vi "angle2DutyCycle.vi"(1 "Steering Angle":dbl min=-21.0 max=21.0 step=1.0) -> (0 "Duty Cycle":dbl)   [LabVIEW 2016]
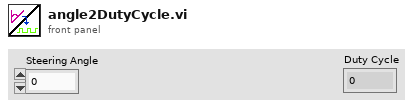
[diagram p1: front panel]
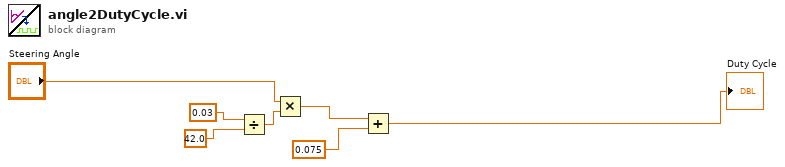
[diagram p0: block diagram]
diagram:
  n1 = Divide(x=0.03, y=42.0) -> (x/y=w5:dbl)
  n2 = Multiply(x="Steering Angle", y=w5) -> (x*y=w3:dbl)
  n3 = Add(x=w3, y=0.075) -> (x+y=→"Duty Cycle":dbl)
